vi "FitGaussian3(SubVI).vi"(0 "x values":dbl[](array[numeric])=[13.399933, 13.44983225, 13.5001315, 13.55013075, 13.59993, 13.65002925, 13.7001285, 13.75002775, 13.800127, 13.84992625, 13.9000255, 13.95002475, 13.999924, 14.0500207, 14.1000174, 14.1499141, 14.2001108, 14.2500075, 14.2998042, 14.3501009, 14.3999976, 14.4497943, 14.499991, 14.5498877, 14.6000844, 14.6499811, 14.6997778, 14.7500745, 14.8000712, 14.8498679, 14.8999646, 14.9500613, 14.999958, 15.0501404, 15.1001228, 15.1501052, 15.2002876, 15.25017, 15.3001524, 15.3502348, 15.4000172, 15.4501996, 15.500082, 15.5498644, 15.6002468, 15.6502292, 15.6999116, 15.750094, 15.8001764, 15.8498588, 15.9001412, 15.9500236, 15.999906, 16.05021475, 16.0999235, 16.15003225, 16.200241, 16.25004975, 16.3000585, 16.34996725, 16.399876, 16.45018475, 16.5001935, 16.54990225], 1 "y values":dbl[](array[numeric])=[42.648277282714844, 43.9074821472168, 44.95804977416992, 46.04310607910156, 46.7999382019043, 47.876556396484375, 48.90898513793945, 49.69123077392578, 50.29452896118164, 50.99095153808594, 51.3321533203125, 52.05470657348633, 52.37543869018555, 52.83419418334961, 53.5294303894043, 53.09951400756836, 52.98366928100586, 52.9737663269043, 52.82147216796875, 52.25721740722656, 51.93815612792969, 50.699134826660156, 50.42073440551758, 49.25381088256836, 48.3885383605957, 47.47373580932617, 46.43144226074219, 45.583709716796875, 43.905120849609375, 42.53858184814453, 41.602542877197266, 40.06209182739258, 39.04403305053711, 37.436161041259766, 36.6154899597168, 35.539791107177734, 34.32120132446289, 33.28242874145508, 32.38603210449219, 31.3276309967041, 30.748254776000977, 29.91518783569336, 29.445737838745117, 28.354888916015625, 28.009984970092773, 27.285934448242188, 27.04413414001465, 26.576818466186523, 25.898874282836914, 25.55618667602539, 25.26278305053711, 24.908693313598633, 25.03961753845215, 24.513620376586914, 24.64219093322754, 25.168533325195312, 24.8322811126709, 25.24604606628418, 25.068620681762695, 25.58075714111328, 25.197729110717773, 25.184911727905273, 25.455291748046875, 25.335906982421875], 2 "delta y values":dbl[](array[numeric])=[1.0, 1.0, 1.0, 1.0, 1.0, 1.0, 1.0, 1.0, 1.0, 1.0, 1.0, 1.0, 1.0, 1.0, 1.0, 1.0, 1.0, 1.0, 1.0, 1.0, 1.0, 1.0, 1.0, 1.0, 1.0, 1.0, 1.0, 1.0, 1.0, 1.0, 1.0, 1.0, 1.0, 1.0, 1.0, 1.0, 1.0, 1.0, 1.0, 1.0, 1.0, 1.0, 1.0, 1.0, 1.0, 1.0, 1.0, 1.0, 1.0, 1.0, 1.0, 1.0, 1.0, 1.0, 1.0, 1.0, 1.0, 1.0, 1.0, 1.0, 1.0, 1.0, 1.0, 1.0], 5 "error in":errorcluster, 6 "Fit type":T2=enum."Expect maximum", 7 "confidence level":dbl=0.95, 12 "Minimization inputs":T4={"Minimizing alg"=0, "Search accuracy"=1e-08, "Step type"=0} {"Step type" items=["fixed function", "modified function"]; "Search accuracy" format="%.2e"; "Minimizing alg" items=["Golden Section Search", "Brent with Derivatives"]}) -> (14 "Plot":T5, 15 "Optimized position":dbl, 16 "Uncertainty on position":dbl, 17 "standard deviation":dbl, 18 "delta standard deviation":dbl, 19 "error out":errorcluster)   [LabVIEW 2016]
uses:
  Utils/Controls/Graph_TypeDef_XY.ctl
  Utils/Controls/All_Enums/Enum_TypeDef_ParabolaFitType.ctl
  <vilib>/Analysis/6fits.llb/Curve Fitting Criteria.ctl
  <vilib>/Analysis/6fits.llb/Confidence Interval (Gauss).vi
  <vilib>/gmath/NI_Gmath.lvlib
  <vilib>/Analysis/NI_AALPro.lvlib
panel:
  out "Y error bars":cluster{dbl[], dbl[]}(graph)
  in  "Tab Control":T1(tab)
  in  "method":T3 items=["Least Square", "Least Absolute Residual", "Bisquare"]
  out "amplitude":dbl
  out "center":dbl
  out "delta center":dbl
  out "delta amplitude":dbl
  out "Fitted quadratic":string
  out "f(optimized position)":dbl[](array[numeric]) format="%.2f"
  out "Best Gaussian Fit":dbl[](array[numeric])
  out "Fit residue":dbl
  out "Polynomial Coefficients":dbl[](array[numeric])
  # "FIT Gaussian 3 Brandeis University - Brookhaven National Laboratory * ATLAS Phase II Inner Tracker Upgrade"
  # "-(formula) if looking for a maxium instead"
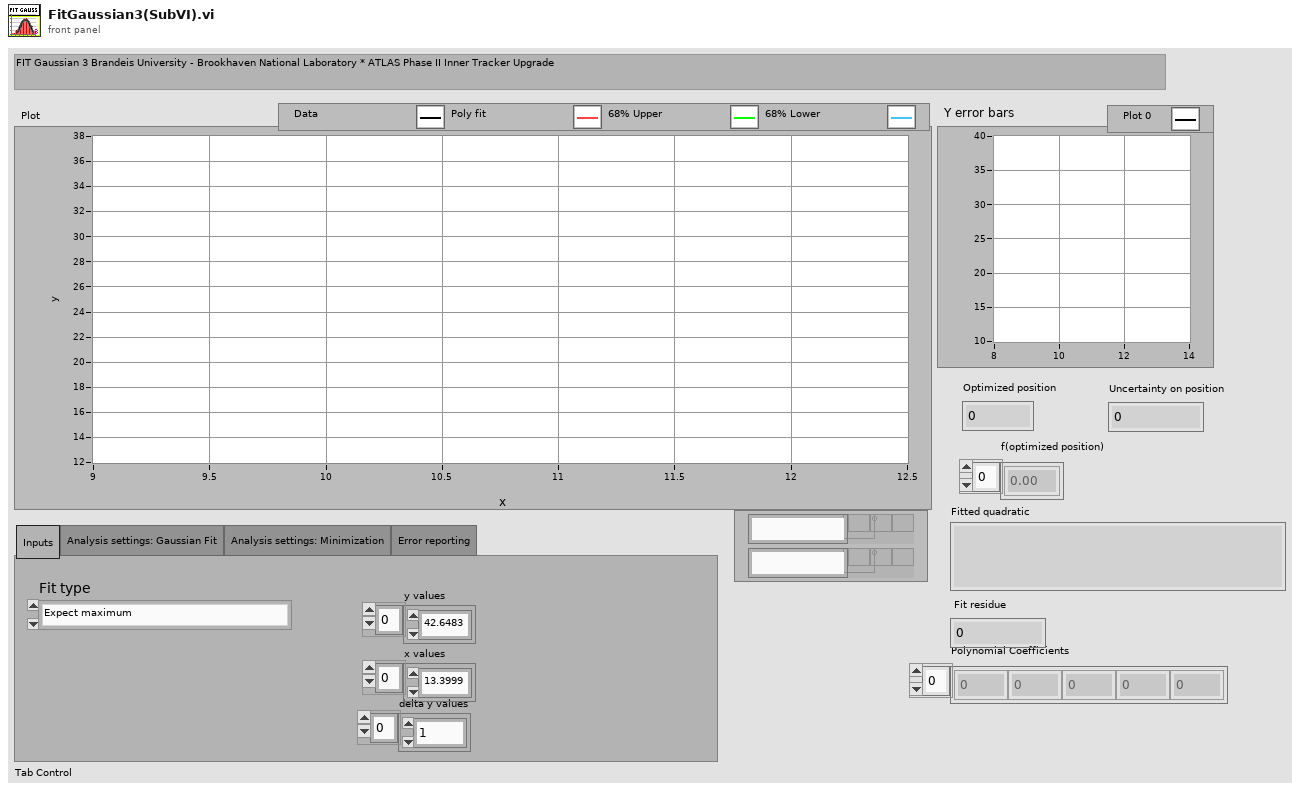
[diagram p1: front panel]
types:
  T1 = enum32{"Inputs", "Analysis settings: Gaussian Fit", "Analysis settings: Minimization", "Error reporting"}
  T2 = typedef "Enum_TypeDef_ParabolaFitType.ctl" = enum16{"Expect minimum", "Expect maximum"}
  T3 = typedef "NI_AALPro.lvlib/Curve Fitting Criteria.ctl" = u16
  T4 = cluster{"Minimizing alg":u16, "Search accuracy":dbl, "Step type":u16}
  T5 = typedef "Graph_TypeDef_XY.ctl" = cluster{"Radius bins":dbl[], "Best Gaussian Fit":dbl[]}[]
  T6 = typedef "Enum_TypeDef_Tails.ctl" = enum16{"No tails", "Left tail", "Right tail"}
  T7 = cluster{"Selected x values":dbl[], "Best Gaussian Fit":dbl[]}
  T8 = cluster{"Selected x values":dbl[], "Upper Bound":dbl[]}
  T9 = cluster{"Selected x values":dbl[], "Lower Bound":dbl[]}
  T10 = cluster{"Selected x values":dbl[], "Lower Bound":dbl[]}[]
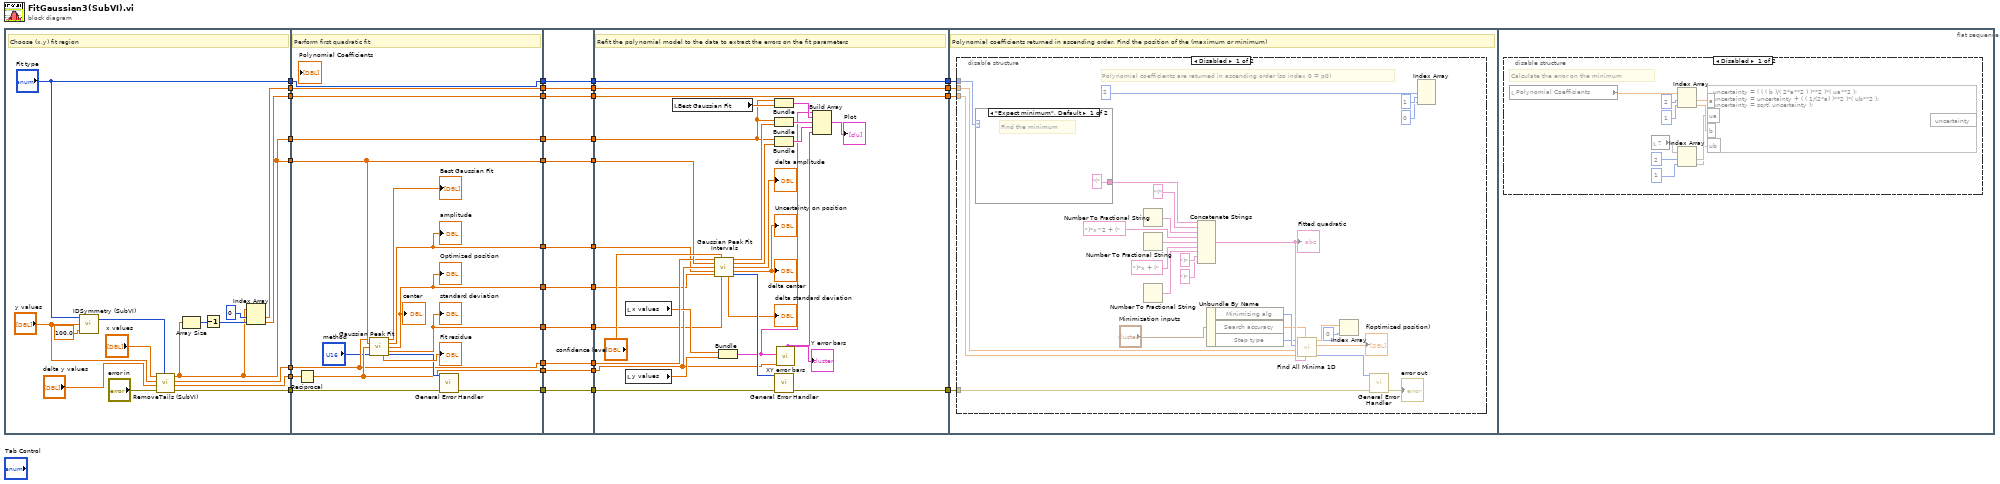
[diagram p0: block diagram]
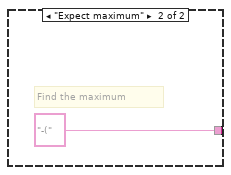
[diagram p2: hidden frame]
diagram:
  n1 = flat-sequence {
    tunnel: [w43] -> w33
    tunnel: [w41] -> w32
    tunnel: [w42] -> w31
    tunnel: [w43] -> w30
    tunnel: [w47] -> w29
    tunnel: [w46] -> w28
    tunnel: ["Fit type"] -> w25
    tunnel: [w35] -> w7
    tunnel: [w65] -> w23
    tunnel: w33 -> [w63]
    tunnel: w32 -> [w64]
    tunnel: w31 -> [w56]
    tunnel: [w63] -> w21
    tunnel: [w56] -> w19
    tunnel: [w58] -> w17
    tunnel: w30 -> [w62]
    tunnel: [w62] -> w15
    tunnel: w29 -> [w61]
    tunnel: w28 -> [w60]
    tunnel: [w61] -> w13
    tunnel: [w60] -> w11
    tunnel: w25 -> [w59]
    tunnel: [w59] -> w9
    tunnel: w7 -> [w55]
    tunnel: [w51] -> w6
    tunnel: [w53] -> w4
    tunnel: [w52] -> w2
    tunnel: w23 -> [w78]
    tunnel: [w78] -> w22
    tunnel: w21 -> [w77]
    tunnel: [w77] -> w20
    tunnel: w19 -> [w76]
    tunnel: [w76] -> w18
    tunnel: w17 -> [w75]
    tunnel: [w75] -> w16
    tunnel: w15 -> [w74]
    tunnel: [w74] -> w14
    tunnel: w13 -> [w73]
    tunnel: [w73] -> w12
    tunnel: w11 -> [w72]
    tunnel: [w72] -> w10
    tunnel: w9 -> [w71]
    tunnel: [w71] -> w8
    tunnel: w6 -> [w70]
    tunnel: [w70] -> w5
    tunnel: w4 -> [w69]
    tunnel: [w69] -> w3
    tunnel: w2 -> [w68]
    tunnel: [w68] -> w1
    tunnel: w22 -> [w97]
    tunnel: [w96] -> w34
    tunnel: w20 -> [w95]
    tunnel: w18 -> [w94]
    tunnel: w16 -> [w87]
    tunnel: w14 -> [w93]
    tunnel: w12 -> [w89]
    tunnel: w10 -> [w88]
    tunnel: [w89] -> w27
    tunnel: [w88] -> w26
    tunnel: [w86] -> w24
    tunnel: w8 -> [w86]
    tunnel: w5 -> [w82]
    tunnel: w3 -> [w81]
    tunnel: w1 -> [w80]
    tunnel: w34 -> [w110]
    tunnel: w27 -> [w109]
    tunnel: w26 -> [w108]
    tunnel: w24 -> [w107]
    frame #0 {
      # "Choose (x,y) fit region"
      n2 = call "IDSymmetry (SubVI).vi"("Tolerance (%)"=100.0, "Values"="y values", "Fit type"="Fit type") -> ("Side of Tail"=w38:T6)  [unwired: 1 out]
      n3 = call "RemoveTails (SubVI).vi"("Side of Tail"=w38, "error in (no error)"="error in", "delta y values"="delta y values", "y values"="y values", "x values"="x values") -> ("error out"=w35:errorcluster, "Selected delta y values"=w41:dbl[], "Selected y values"=w42:dbl[], "Selected x values"=w43:dbl[])  [unwired: 3 in]
      n4 = Array Size(array=w43) -> (size(s)=w49:i32)
      n5 = Decrement(x=w49) -> (x-1=w50:i32)
      n6 = Index Array(array=w43, index #1=0 ("index"), index #2=w50) -> (element #1=w47:dbl, element #2=w46:dbl)
    }
    frame #1 {
      # "Perform first quadratic fit"
      n7 = Reciprocal(x=w64) -> (1/x=w58:dbl[])
      n8 = call <vilib>:"Gaussian Peak Fit.vi"("Y"=w56, "X"=w63, "Weight"=w58, "method"="method") -> ("Best Gaussian Fit"=→"Best Gaussian Fit":dbl[], "amplitude"=w53:dbl, "center"=w51:dbl, "standard deviation"=w52:dbl, "residue"=→"Fit residue":dbl, "error"=w66:i32)  [unwired: 5 in, 1 out]
      "amplitude" <- w53
      "center" <- w51
      "standard deviation" <- w52
      "Optimized position" <- w51
      n9 = call <vilib>:"General Error Handler.vi"("[error code] (0)"=w66, "error in (no error)"=w55) -> ("error out"=w65:errorcluster)  [unwired: 9 in, 4 out]
    }
    frame #2 {
    }
    frame #3 {
      # "Refit the polynomial model to the data to extract the errors on the fit parameters"
      n10 = local read "x values"() -> (w92:dbl[])
      n11 = local read "y values"() -> (w105:dbl[])
      n12 = local read "Best Gaussian Fit"() -> (w104:dbl[])
      n13 = call-poly <vilib>:"Gaussian Peak Fit Intervals.vi"("Y"=w94, "confidence level"="confidence level", "X"=w95, "Weight"=w87, "amplitude"=w81, "center"=w82, "standard deviation"=w80) -> ("Upper Bound"=w103:dbl[], "Lower Bound"=w102:dbl[], "delta amplitude"=→"delta amplitude":dbl, "delta center"=→"delta center" →"Uncertainty on position":dbl, "delta standard deviation"=→"delta standard deviation":dbl, "error"=w98:i32)  [unwired: 3 in]
      n14 = Bundle("x values"=w92, "y values"=w105) -> (w90:cluster{"x values":dbl[], "y values":dbl[]})  [unwired: 1 in]
      n15 = Bundle("Selected x values"=w93, "Best Gaussian Fit"=w104) -> (w101:T7)  [unwired: 1 in]
      n16 = Bundle("Selected x values"=w93, "Upper Bound"=w103) -> (w100:T8)  [unwired: 1 in]
      n17 = Bundle("Selected x values"=w93, "Lower Bound"=w102) -> (w99:T9)  [unwired: 1 in]
      n18 = call <vilib>:"General Error Handler.vi"("[error code] (0)"=w98, "error in (no error)"=w97) -> ("error out"=w96:errorcluster)  [unwired: 9 in, 4 out]
      n19 = call "XY error bars.vi"("XY plot"=w90, "Yerror"=w87) -> ("Y error bars"=w85:cluster{dbl[], dbl[]})  [unwired: 6 in, 2 out]
      "Y error bars" <- w85
      n20 = Build Array(w90, w101, w100, w99, w85) -> (→"Plot":T10)
    }
    frame #4 {
      # "Polynomial coefficients returned in ascending order. Find the position of the (maximum or minimum)"
      n21 = disable-structure shown="Disabled" {
        disable-tunnel: w110 -> [w123 _]
        disable-tunnel: w109 -> [w116 _]
        disable-tunnel: w108 -> [w115 _]
        disable-tunnel: w107 -> [w114 _]
        frame Disabled {
          # "Polynomial coefficients are returned in ascending order (so index 0 = p0)"
          n22 = case shown="\"Expect minimum\", Default" w114 {
            tunnel: ["(" "-("] -> w118
            frame "Expect minimum", Default {
              # "Find the minimum"
            }
            frame "Expect maximum" {
              # "Find the maximum"
            }
          }
          n23 = Number To Fractional String() -> (F-format string=w131:string)  [unwired: 4 in]
          n24 = Number To Fractional String() -> (F-format string=w130:string)  [unwired: 4 in]
          n25 = Number To Fractional String() -> (F-format string=w129:string)  [unwired: 4 in]
          n26 = Concatenate Strings(w118, "(" ("string"), w131, ")*x^2 + (" ("string"), w130, ")*x + (" ("string"), w129, ")" ("string"), ")" ("string")) -> (w136:string)
          "Fitted quadratic" <- w136
          n27 = Unbundle By Name("Minimization inputs") -> ("Minimizing alg"=w122:u16, "Search accuracy"=w121:dbl, "Step type"=w120:u16)
          n28 = call <vilib>:"Find All Minima 1D.vi"("formula"=w136, "accuracy"=w121, "end"=w115, "start"=w116, "algorithm"=w122, "step type"=w120) -> ("error"=w125:i32, "f(Minima)"=→"f(optimized position)":dbl[], "Minima"=w113:dbl[])  [unwired: 1 out]
          n29 = Index Array(array=w113, index=0) -> (element=w111:dbl)
          n30 = call <vilib>:"General Error Handler.vi"("[error code] (0)"=w125, "error in (no error)"=w123) -> ("error out"=→"error out":errorcluster)  [unwired: 9 in, 4 out]
          n31 = Index Array(index #1=2 ("index"), index #2=1 ("index"), index #3=0 ("index")) -> ()  [unwired: 1 in, 3 out]
        }
        frame Enabled {
        }
      }
    }
    frame #5 {
      n32 = disable-structure shown="Disabled" {
        frame Disabled {
          # "Calculate the error on the minimum"
          n33 = local read "Polynomial Coefficients"() -> (w146:dbl[])
          n34 = local read item#-1() -> (w149)
          n35 = Index Array(array=w146, index #1=2 ("index"), index #2=1 ("index")) -> (element #1=w143:dbl, element #2=w142:dbl)
          n36 = Index Array(array=w149, index #1=2 ("index"), index #2=1 ("index")) -> (element #1=w141, element #2=w140)
          n37 = formula code="uncertainty = ( ( ( b )/( 2*a**2 ) )**2 )*( ua**2 );\nuncertainty = uncertainty + ( ( 1/(2*a) )**2 )*( ub**2 ); \nuncertainty = sqrt( uncertainty );"("a"=w143, "b"=w142, "ua"=w141, "ub"=w140) -> ()  [unwired: 1 out]
        }
        frame Enabled {
        }
      }
    }
  }
